vi "Z6CSMain.panel.vi"(0 "object ref":refnum<vi>, 5 "error in (no error)":errorcluster) -> (19 "error out":errorcluster)   [LabVIEW 2014, in "Z6CSMain.lvlib"]
doc: "This is just an example for a GUI thread.\n\nLicense Agreement for this software:\n\nCopyright (C)\nGesellschaft für Schwerionenforschung, GSI\nPlanckstr. 1\n64291 Darmstadt\nGermany\n\nContact: D.Beck@gsi.de \n\nThis program is free software; you can redistribute it and/or modify it under the terms of the GNU General Public License as published by the Free Software Foundation; either version 2 of the license, or (at your option) any later version.\n\nThis program is distributed in the hope that it will be useful, but WITHOUT ANYW ARRANTY; without even the implied warranty of MERCHANTABILITY or FITNESS FOR A PARTICULAR PURPOSE. See the GNU General License for more details (http://www.gnu.org).\n\nGesellschaft für Schwerionenforschung, GSI\nPlanckstr. 1, 64291 Darmstadt, Germany\nFor all questions and ideas contact: M.Richter@gsi.de, H.Brand@gsi.de or D.Beck@gsi.de.\nLast update: 18-DEC-2002"
uses:
  Z6CSMain.lvlib
  CS_Core/CSObj/CSObj.lvlib
  PH_Basics/PH_Common/PH_Common.lvlib
  PCSMain/PCSMain.lvlib
panel:
  in  "VISA":bool
  in  "Powermeter Statistician":bool
  in  "Powermeter List":bool
  in  "SHS Anal Statistician":bool
  in  "SHS Analyzer":bool
  in  "SHS Analysis Calibrator":bool
  in  "Remote Desktop Connection":bool
  in  "Minimize":bool
  in  "Beckhoff Watch Dog":bool
  in  "Countdown":bool
  in  "Seq Watch":bool
  in  "Vacuum Controllers":bool
  in  "SSAC":bool
  in  "Switch List":bool
  in  "BB List":bool
  in  "Spectrometer":bool
  in  "Z6 Beamline":bool
  in  "6P List":bool
  in  "Scopes":bool
  in  "Current Meas":bool
  in  "Calorimeter":bool
  in  "Cam List":bool
  in  "PCS System Indicator":bool caption="PCS"
  in  "Fast CoG":bool
  in  "Image Statistician":bool
  in  "Powermeter":bool
  in  "DataViewer":bool
  in  "Beamline":bool
  out "stopped":bool
  in  "BlackBoxes":bool
  in  "Operators":bool
  in  "Calibrator":bool
  in  "GateDelayGens":bool
  in  "Switch GUIs":bool
  in  "Motion GUIs":bool
  in  "Cameras":bool
  in  "Sequencer":bool
  in  "Delete":bool
  out "loop counter":i32
  # "Z6-CS"
  # "3.40"
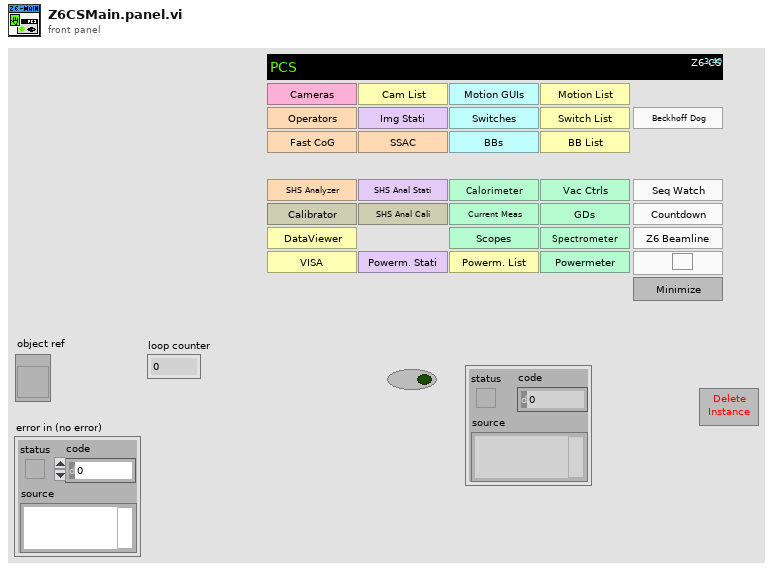
[diagram p1: front panel]
types:
  T1 = enum16{"None", "PCS Main", "Z6 Main", "PCS Beamline", "Z6 Beamline", "Image Statistician", "Powermeter Statistician", "SHS Anal Statistician", "Image Center of Gravity", "Image Calibrator", "SHS Analysis Calibrator"}
  T2 = enum16{"None", "PCS Main", "Z6 Main", "PCS Beamline", "Z6 Beamline", "Image Statistician", "Powermeter Statistician", "SHS Anal Statistician", "Image Center of Gravity", "Image Calibrator", "SHS Analysis Calibrator", "Cam List", "Powermeterlist", "6P List", "BB List", "Switch List", "Sequence Watch"}
  T3 = typedef "PCSMain.lvlib/PCSMain.i attribute.ctl" = cluster{"System Objects":cluster{"Spectrometer Objects":string[], "Camera Objects":string[], "Image Operator Objects":string[], "Gate- and Delaygenerators":string[], "Current Meas Objects":string[], "Calorimeter Objects":string[], "Powermeter Objects":string[], "SSAC Objects":string[], "Vacuum Control Objects":string[], "Countdown Counter Objects":string[], "Beckhoff Watchdog Objects":string[], "SHS Analyzer Objects":string[]}, "Local Objects":cluster{"Spectrometer Objects":string[], "Camera Objects":string[], "Image Operator Objects":string[], "Gate- and Delaygenerators":string[], "Current Meas Objects":string[], "Calorimeter Objects":string[], "Powermeter Objects":string[], "SSAC Objects":string[], "Vacuum Control Objects":string[], "Countdown Counter Objects":string[], "Beckhoff Watchdog Objects":string[], "SHS Analyzer Objects":string[]}, "Systems on same node":string[], "Data Viewer visible?":bool, "Running Objects":cluster{"Operators":bool, "SHS Analyzers":bool}, "Cam Instance System ID":string, "Black Box Objects":string[], "Switch Objects":string[], "Motion GUI Objects":string[], "Osci Objects":string[]}
  T4 = enum16{"PCS", "Laser", "Vision", "PP", "Special", "Beckhoff"}
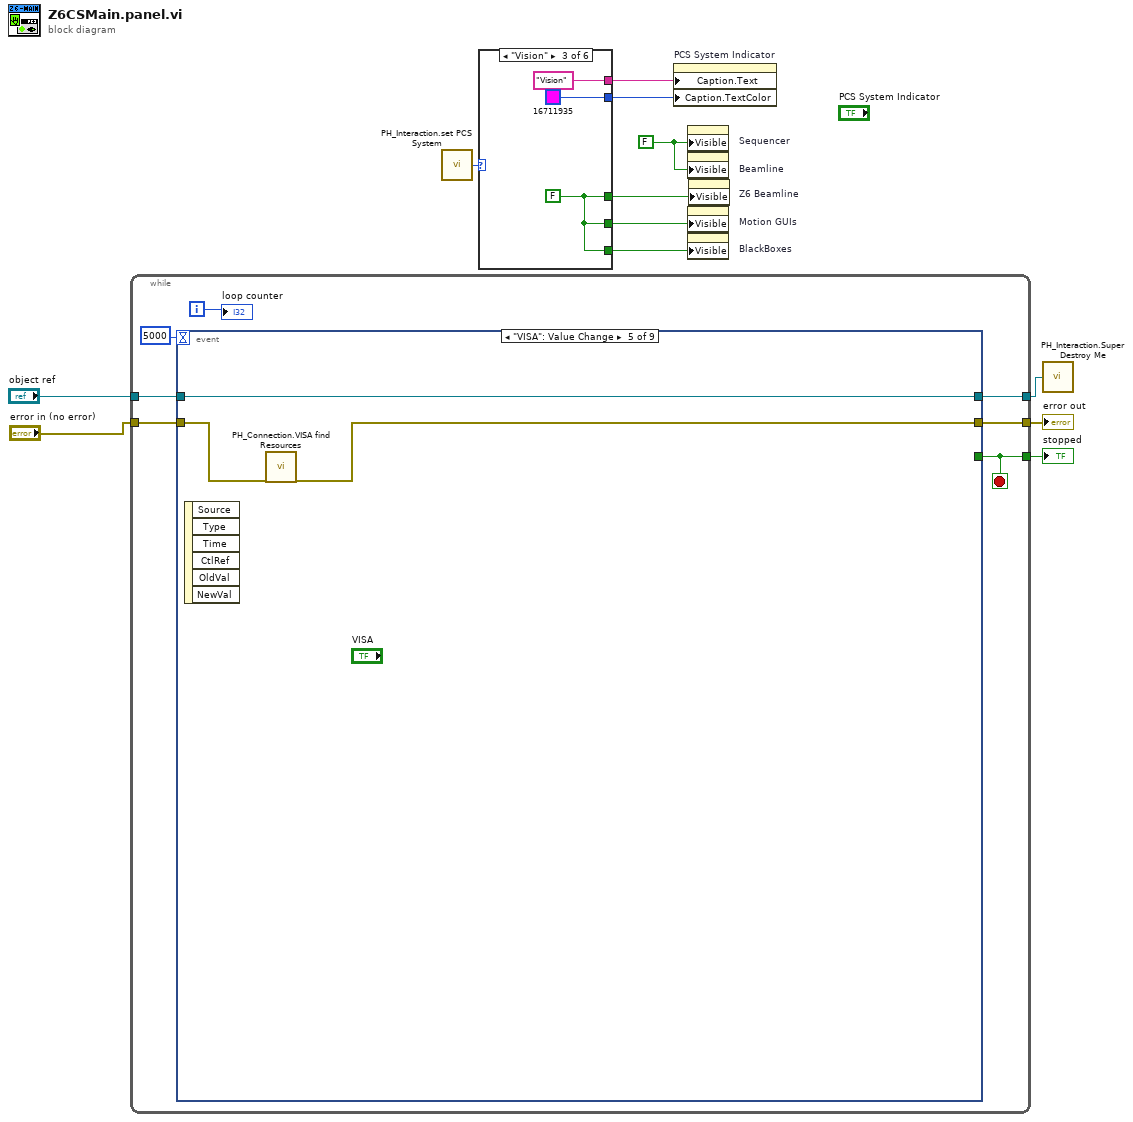
[diagram p0: block diagram]
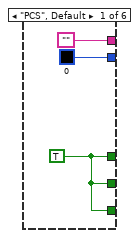
[diagram p2: hidden frame]
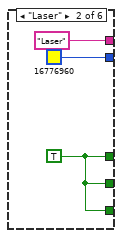
[diagram p3: hidden frame]
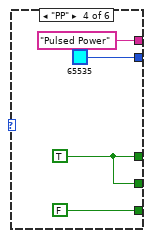
[diagram p4: hidden frame]
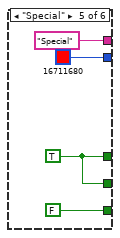
[diagram p5: hidden frame]
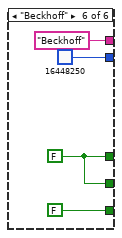
[diagram p6: hidden frame]
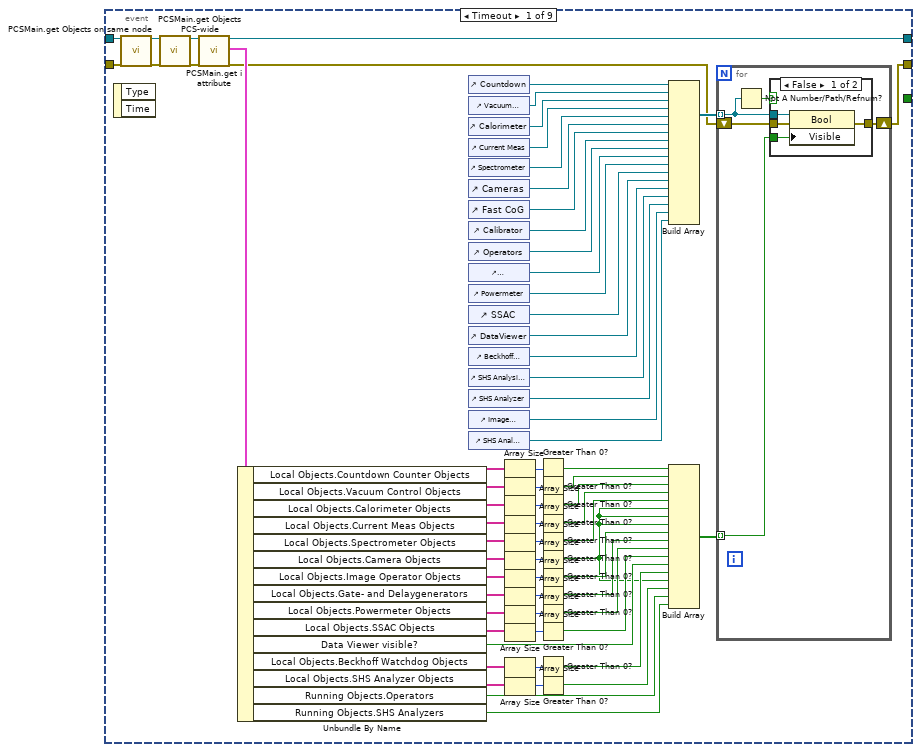
[diagram p7: hidden frame]
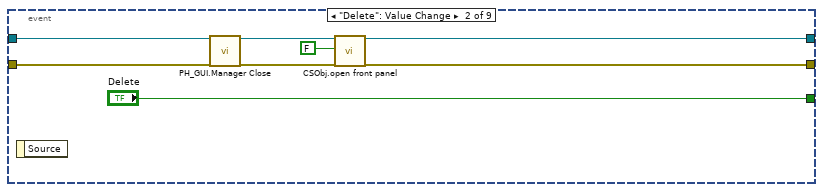
[diagram p9: hidden frame]
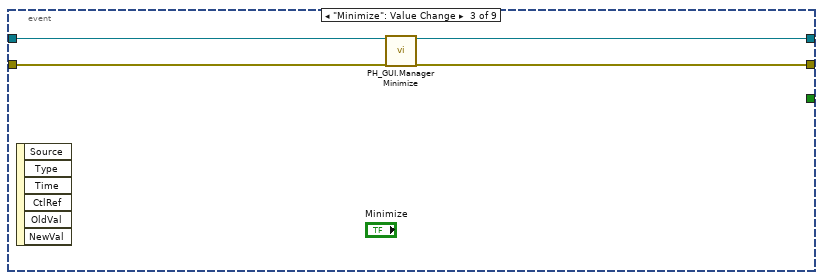
[diagram p10: hidden frame]
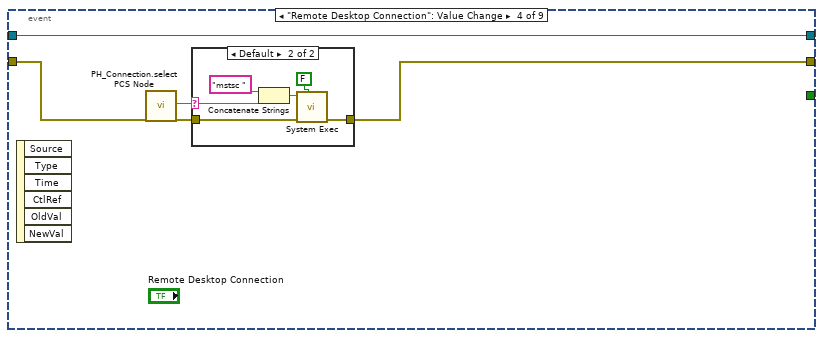
[diagram p11: hidden frame]
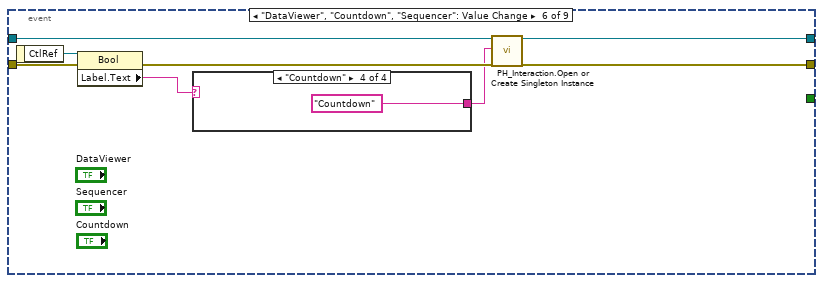
[diagram p13: hidden frame]
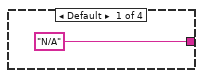
[diagram p14: hidden frame]
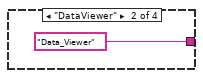
[diagram p15: hidden frame]
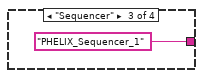
[diagram p16: hidden frame]
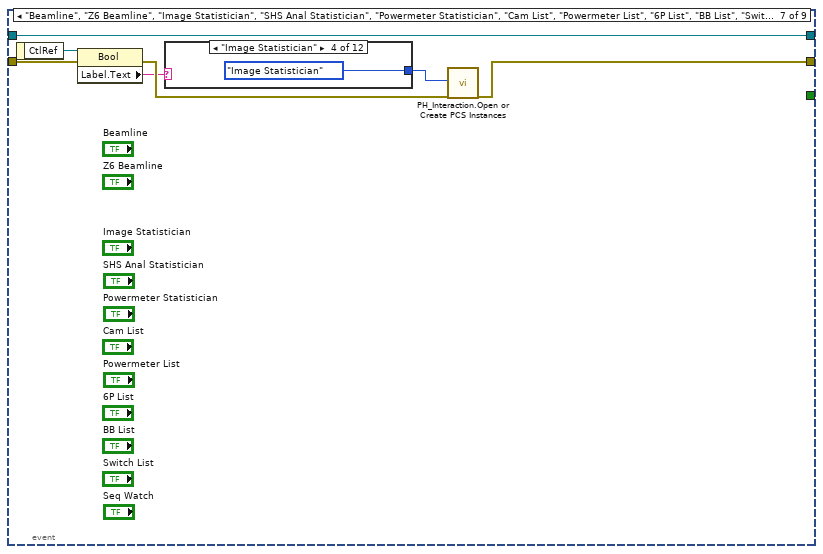
[diagram p17: hidden frame]
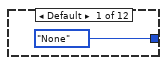
[diagram p18: hidden frame]
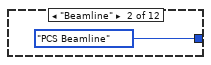
[diagram p19: hidden frame]
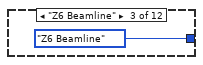
[diagram p20: hidden frame]
diagram:
  w1 = FALSE
  n1 = while {
    tunnel: "object ref" -> [w15]
    tunnel: [w14] -> w10
    tunnel: [w18] -> w11
    tunnel: "error in (no error)" -> [w17]
    tunnel: [w16] -> w12
    i -> [w19]
    stop <- w16 stop-if-true
    n2 = event shown="[4] \"VISA\": Value Change" {
      selector: _ -> [_ _ _ _ _ _ _ _ _]
      dyn-events: _ -> [_ _ _ _ _ _ _ _ _]
      timeout: 5000 -> [_ _ _ _ _ _ _ _ _]
      tunnel: w15 -> [w87 w104 w110 w114 w125 w128 w141 w164 w182]
      tunnel: [_ "Delete" _ _ _ _ _ _ _] -> w16
      tunnel: [w62 w103 w107 w112 w123 w129 w144 w167 w180] -> w18
      tunnel: w17 -> [w88 w100 w109 w115 w124 w132 w142 w165 w181]
      tunnel: [w61 w102 w108 w114 w125 w127 w141 w163 w176] -> w14
      event Timeout {
        n3 = event-data() -> ()  [unwired: 1 in, 2 out]
        n4 = call "PCSMain.get Objects on same node.vi"("i ref in"=w87, "error in (no error)"=w88) -> ("i ref out"=w23:refnum<vi>, "error out"=w21:errorcluster)  [unwired: 16 in]
        n5 = call "PCSMain.get Objects PCS-wide.vi"("i ref in"=w23, "error in (no error)"=w21) -> ("i ref out"=w22:refnum<vi>, "error out"=w20:errorcluster)  [unwired: 16 in]
        n6 = call "PCSMain.get i attribute.vi"("i ref in"=w22, "error in (no error)"=w20) -> ("i ref out"=w61:refnum<vi>, "i attribute"=w86:T3, "error out"=w63:errorcluster)  [unwired: 15 in]
        n7 = Unbundle By Name(w86) -> ("Local Objects.Countdown Counter Objects"=w43:string[], "Local Objects.Vacuum Control Objects"=w47:string[], "Local Objects.Calorimeter Objects"=w82:string[], "Local Objects.Current Meas Objects"=w75:string[], "Local Objects.Spectrometer Objects"=w73:string[], "Local Objects.Camera Objects"=w71:string[], "Local Objects.Image Operator Objects"=w70:string[], "Local Objects.Gate- and Delaygenerators"=w68:string[], "Local Objects.Powermeter Objects"=w66:string[], "Local Objects.SSAC Objects"=w38:string[], "Data Viewer visible?"=w49:bool, "Local Objects.Beckhoff Watchdog Objects"=w40:string[], "Local Objects.SHS Analyzer Objects"=w30:string[], "Running Objects.Operators"=w25:bool, "Running Objects.SHS Analyzers"=w24:bool)
        n8 = control-ref of="Countdown"() -> (w44:refnum<vi>)
        n9 = control-ref of="Vacuum Controllers"() -> (w48:refnum<vi>)
        n10 = control-ref of="Calorimeter"() -> (w60:refnum<vi>)
        n11 = control-ref of="Current Meas"() -> (w59:refnum<vi>)
        n12 = control-ref of="Spectrometer"() -> (w58:refnum<vi>)
        n13 = control-ref of="Cameras"() -> (w57:refnum<vi>)
        n14 = control-ref of="Fast CoG"() -> (w53:refnum<vi>)
        n15 = control-ref of="Calibrator"() -> (w52:refnum<vi>)
        n16 = control-ref of="Operators"() -> (w56:refnum<vi>)
        n17 = control-ref of="GateDelayGens"() -> (w55:refnum<vi>)
        n18 = control-ref of="Powermeter"() -> (w54:refnum<vi>)
        n19 = control-ref of="SSAC"() -> (w51:refnum<vi>)
        n20 = control-ref of="DataViewer"() -> (w50:refnum<vi>)
        n21 = control-ref of="Beckhoff Watch Dog"() -> (w35:refnum<vi>)
        n22 = control-ref of="SHS Analysis Calibrator"() -> (w33:refnum<vi>)
        n23 = control-ref of="SHS Analyzer"() -> (w28:refnum<vi>)
        n24 = control-ref of="Image Statistician"() -> (w27:refnum<vi>)
        n25 = control-ref of="SHS Anal Statistician"() -> (w26:refnum<vi>)
        n26 = Array Size(array=w43) -> (size(s)=w41:i32)
        n27 = Array Size(array=w47) -> (size(s)=w45:i32)
        n28 = Array Size(array=w82) -> (size(s)=w83:i32)
        n29 = Array Size(array=w75) -> (size(s)=w80:i32)
        n30 = Array Size(array=w73) -> (size(s)=w79:i32)
        n31 = Array Size(array=w71) -> (size(s)=w78:i32)
        n32 = Array Size(array=w70) -> (size(s)=w77:i32)
        n33 = Array Size(array=w68) -> (size(s)=w76:i32)
        n34 = Array Size(array=w66) -> (size(s)=w64:i32)
        n35 = Array Size(array=w38) -> (size(s)=w37:i32)
        n36 = Array Size(array=w40) -> (size(s)=w39:i32)
        n37 = Array Size(array=w30) -> (size(s)=w31:i32)
        n38 = Greater Than 0?(x=w41) -> (x > 0?=w42:bool)
        n39 = Greater Than 0?(x=w45) -> (x > 0?=w46:bool)
        n40 = Greater Than 0?(x=w83) -> (x > 0?=w81:bool)
        n41 = Greater Than 0?(x=w80) -> (x > 0?=w74:bool)
        n42 = Greater Than 0?(x=w79) -> (x > 0?=w72:bool)
        n43 = Greater Than 0?(x=w78) -> (x > 0?=w32:bool)
        n44 = Greater Than 0?(x=w77) -> (x > 0?=w69:bool)
        n45 = Greater Than 0?(x=w76) -> (x > 0?=w67:bool)
        n46 = Greater Than 0?(x=w64) -> (x > 0?=w65:bool)
        n47 = Greater Than 0?(x=w37) -> (x > 0?=w36:bool)
        n48 = Greater Than 0?(x=w39) -> (x > 0?=w34:bool)
        n49 = Greater Than 0?(x=w31) -> (x > 0?=w29:bool)
        n50 = Build Array(w44, w48, w60, w59, w58, w57, w53, w52, w56, w55, w54, w51, w50, w35, w33, w28, w27, w26) -> (w85:refnum<vi>[])
        n51 = Build Array(w42, w46, w81, w74, w72, w32, w32, w32, w69, w67, w65, w36, w49, w34, w32, w29, w25, w24) -> (w84:bool[])
        n52 = for {
          tunnel: w84 -> [w89] mode=indexing
          tunnel: w85 -> [w92] mode=indexing
          shift-right: [w91] -> w62
          shift-left: w63 -> [w90]
          n53 = Not A Number/Path/Refnum?(number/path/refnum=w92) -> (NaN/Path/Refnum?=w93:bool)
          n54 = case shown="False" w93 {
            tunnel: w89 -> [w97 _]
            tunnel: w92 -> [w96 _]
            tunnel: w90 -> [w95 w98]
            tunnel: [w94 w98] -> w91
            frame False {
              n55 = property class="Bool"(reference=w96, error in=w95, "Visible"=w97) -> (error out=w94:errorcluster)  [unwired: 1 out]
            }
            frame True {
            }
          }
        }
      }
      event "Delete": Value Change {
        n56 = event-data() -> ()  [unwired: 1 in, 1 out]
        n57 = call "PH_GUI.Manager Close.vi"("i ref in"=w104, "error in"=w100) -> ("i ref out"=w101:refnum<vi>, "error out"=w99:errorcluster)  [unwired: 16 in]
        n58 = call "CSObj.open front panel.vi"("i ref in"=w101, "frontPanelOpen"=FALSE ("front panel open"), "error in (no error)"=w99) -> ("i ref out"=w102:refnum<vi>, "error out"=w103:errorcluster)  [unwired: 15 in]
      }
      event "Minimize": Value Change {
        n59 = event-data() -> ()  [unwired: 1 in, 6 out]
        n60 = call "PH_GUI.Manager Minimize.vi"("i ref in"=w110, "error in"=w109) -> ("i ref out"=w108:refnum<vi>, "error out"=w107:errorcluster)  [unwired: 16 in]
      }
      event "Remote Desktop Connection": Value Change {
        n61 = event-data() -> ()  [unwired: 1 in, 6 out]
        n62 = call "PH_Connection.select PCS Node.vi"("error in"=w115) -> ("string out"=w111:string, "error out"=w113:errorcluster)  [unwired: 17 in]
        n63 = case shown="Default" w111 {
          selector: w111 -> [_ w117]
          tunnel: w113 -> [w116 w119]
          tunnel: [w116 w118] -> w112
          frame "", "N/A" {
          }
          frame Default {
            n64 = Concatenate Strings("mstsc " ("command line"), w117) -> (w121:string)
            n65 = call <vilib>:"System Exec.vi"("wait until completion? (T)"=FALSE, "error in (no error)"=w119, "command line"=w121) -> ("error out"=w118:errorcluster)  [unwired: 5 in, 3 out]
          }
        }
      }
      event "VISA": Value Change {
        n66 = event-data() -> ()  [unwired: 1 in, 6 out]
        n67 = call "PH_Connection.VISA find Resources.vi"("error in"=w124) -> ("error out"=w123:errorcluster)  [unwired: 17 in, 1 out]
      }
      event "DataViewer", "Countdown", "Sequencer": Value Change {
        n68 = event-data() -> ("CtlRef"=w133:refnum<vi>)  [unwired: 1 in]
        n69 = property class="Bool"(reference=w133, error in=w132) -> (error out=w130:errorcluster, "Label.Text"=w131:string)  [unwired: 1 out]
        n70 = case shown="\"Countdown\"" w131 {
          tunnel: ["N/A" "Data_Viewer" "PHELIX_Sequencer_1" "Countdown"] -> w126
          frame Default {
          }
          frame "DataViewer" {
          }
          frame "Sequencer" {
          }
          frame "Countdown" {
          }
        }
        n71 = call "PH_Interaction.Open or Create Singleton Instance.vi"("i ref in"=w128, "Instance to create or to open"=w126, "error IO"=w130) -> ("i ref out"=w127:refnum<vi>, "error out"=w129:errorcluster)  [unwired: 15 in]
      }
      event "Beamline", "Z6 Beamline", "Image Statistician", "SHS Anal Statistician", "Powermeter Statistician", "Cam List", "Powermeter List", "6P List", "BB List", "Switch List", "Seq Watch": Value Change {
        n72 = event-data() -> ("CtlRef"=w143:refnum<vi>)  [unwired: 1 in]
        n73 = property class="Bool"(reference=w143, error in=w142) -> (error out=w140:errorcluster, "Label.Text"=w139:string)  [unwired: 1 out]
        n74 = case shown="\"Image Statistician\"" w139 {
          tunnel: [T1."None" ("Instance to create or open") T1."PCS Beamline" ("Instance to create or open") T1."Z6 Beamline" ("Instance to create or open") T1."Image Statistician" ("Instance to create or open") T1."SHS Anal Statistician" ("Instance to create or open") T1."Powermeter Statistician" ("Instance to create or open") T2."Cam List" ("Instance to create or open") T2."Powermeterlist" ("Instance to create or open") T2."6P List" ("Instance to create or open") T2."BB List" ("Instance to create or open") T2."Switch List" ("Instance to create or open") T2."Sequence Watch" ("Instance to create or open")] -> w138
          frame Default {
          }
          frame "Beamline" {
          }
          frame "Z6 Beamline" {
          }
          frame "Image Statistician" {
          }
          frame "SHS Anal Statistician" {
          }
          frame "Powermeter Statistician" {
          }
          frame "Cam List" {
          }
          frame "Powermeter List" {
          }
          frame "6P List" {
          }
          frame "BB List" {
          }
          frame "Switch List" {
          }
          frame "Seq Watch" {
          }
        }
        n75 = call "PH_Interaction.Open or Create PCS Instances.vi"("Instance to create or open"=w138, "error IO"=w140) -> ("error out"=w144:errorcluster)  [unwired: 17 in]
      }
      event "Calibrator", "SHS Analysis Calibrator", "Fast CoG": Value Change {
        n76 = event-data() -> ("CtlRef"=w166:refnum<vi>)  [unwired: 1 in]
        n77 = property class="Bool"(reference=w166, error in=w165) -> (error out=w162:errorcluster, "Label.Text"=w158:string)  [unwired: 1 out]
        n78 = case shown="\"Fast CoG\"" w158 {
          tunnel: [T1."None" ("Instance to create or open") T1."Image Calibrator" ("Instance to create or open") T1."SHS Analysis Calibrator" ("Instance to create or open") T1."Image Center of Gravity" ("Instance to create or open")] -> w157
          frame Default {
          }
          frame "Calibrator" {
          }
          frame "SHS Analysis Calibrator" {
          }
          frame "Fast CoG" {
          }
        }
        n79 = call "PCSMain.get i attribute.vi"("i ref in"=w164, "error in (no error)"=w162) -> ("i ref out"=w163:refnum<vi>, "i attribute"=w160:T3, "error out"=w161:errorcluster)  [unwired: 15 in]
        n80 = Unbundle By Name(w160) -> ("Cam Instance System ID"=w159:string)
        n81 = call "PH_Interaction.Open or Create PCS Instances.vi"("System ID (N/A)"=w159, "Instance to create or open"=w157, "error IO"=w161) -> ("error out"=w167:errorcluster)  [unwired: 16 in]
      }
      event "Spectrometer", "Cameras", "Operators", "GateDelayGens", "Current Meas", "Calorimeter", "Powermeter", "SSAC", "Vacuum Controllers", "Beckhoff Watch Dog", "SHS Analyzer", "Switch GUIs", "BlackBoxes", "Motion GUIs", "Scopes": Value Change {
        n82 = event-data() -> ("CtlRef"=w178:refnum<vi>)  [unwired: 1 in]
        n83 = property class="Bool"(reference=w178) -> ("Label.Text"=w175:string)  [unwired: 1 in, 2 out]
        n84 = call "PCSMain.get i attribute.vi"("i ref in"=w182, "error in (no error)"=w181) -> ("i ref out"=w177:refnum<vi>, "i attribute"=w174:T3, "error out"=w179:errorcluster)  [unwired: 15 in]
        n85 = case shown="\"Vacuum Controllers\"" w175 {
          tunnel: w174 -> [_ w190 w193 w196 w199 w202 w205 w208 w211 w214 w217 w220 w223 w226 w229 w232]
          tunnel: [string[] [] ("Spectrometer Objects") w189 w191 w194 w197 w200 w204 w207 w210 w213 w216 w219 w222 w225 w228 w231] -> w173
          tunnel: ["N/A" ("Caption.Text") "Spectrometer" ("Caption.Text") "Switch GUIs" ("Caption.Text") "Black Boxes" ("Caption.Text") "Motion GUIs" ("Caption.Text") "Oscilloscopes" ("Caption.Text") "Cameras" ("Caption.Text") "Image Operators" ("Caption.Text") "SHS Analyzers" ("Caption.Text") "Gate and Delay Generators" ("Caption.Text") "Current Measurement" ("Caption.Text") "Calorimeter" ("Caption.Text") "Powermeter" ("Caption.Text") "SSAC" ("Caption.Text") "Vacuum Controller" ("Caption.Text") "Beckhoff Watchdog" ("Caption.Text")] -> w172
          frame Default {
          }
          frame "Spectrometer" {
            n86 = Unbundle By Name(w190) -> ("Local Objects.Spectrometer Objects"=w189:string[])
          }
          frame "Switch GUIs" {
            n87 = Unbundle By Name(w193) -> ("Switch Objects"=w191:string[])
          }
          frame "BlackBoxes" {
            n88 = Unbundle By Name(w196) -> ("Black Box Objects"=w194:string[])
          }
          frame "Motion GUIs" {
            n89 = Unbundle By Name(w199) -> ("Motion GUI Objects"=w197:string[])
          }
          frame "Scopes" {
            n90 = Unbundle By Name(w202) -> ("Osci Objects"=w200:string[])
          }
          frame "Cameras" {
            n91 = Unbundle By Name(w205) -> ("Local Objects.Camera Objects"=w204:string[])
          }
          frame "Operators" {
            n92 = Unbundle By Name(w208) -> ("Local Objects.Image Operator Objects"=w207:string[])
          }
          frame "SHS Analyzer" {
            n93 = Unbundle By Name(w211) -> ("Local Objects.SHS Analyzer Objects"=w210:string[])
          }
          frame "GateDelayGens" {
            n94 = Unbundle By Name(w214) -> ("Local Objects.Gate- and Delaygenerators"=w213:string[])
          }
          frame "Current Meas" {
            n95 = Unbundle By Name(w217) -> ("Local Objects.Current Meas Objects"=w216:string[])
          }
          frame "Calorimeter" {
            n96 = Unbundle By Name(w220) -> ("Local Objects.Calorimeter Objects"=w219:string[])
          }
          frame "Powermeter" {
            n97 = Unbundle By Name(w223) -> ("Local Objects.Powermeter Objects"=w222:string[])
          }
          frame "SSAC" {
            n98 = Unbundle By Name(w226) -> ("Local Objects.SSAC Objects"=w225:string[])
          }
          frame "Vacuum Controllers" {
            n99 = Unbundle By Name(w229) -> ("Local Objects.Vacuum Control Objects"=w228:string[])
          }
          frame "Beckhoff Watch Dog" {
            n100 = Unbundle By Name(w232) -> ("Local Objects.Beckhoff Watchdog Objects"=w231:string[])
          }
        }
        n101 = call "PH_Strings.select string from array.vi"("String Array in"=w173, "Caption.Text"=w172, "error in (no error)"=w179) -> ("string out"=w185:string, "index"=w183:i32, "error out"=w184:errorcluster)  [unwired: 14 in]
        n102 = case shown="-1" w183 {
          tunnel: w184 -> [w234 w239]
          tunnel: [w234 w238] -> w180
          tunnel: w185 -> [_ w237]
          tunnel: w177 -> [w233 w236]
          tunnel: [w233 w235] -> w176
          frame -1 {
          }
          frame Default {
            n103 = call "PH_Interaction.Open or Create Singleton Instance.vi"("i ref in"=w236, "Instance to create or to open"=w237, "error IO"=w239) -> ("i ref out"=w235:refnum<vi>, "error out"=w238:errorcluster)  [unwired: 15 in]
          }
        }
      }
    }
    "loop counter" <- w19
  }
  "error out" <- w11
  "stopped" <- w12
  n104 = call "PH_Interaction.set PCS System.vi"() -> ("Enum"=w9:T4)  [unwired: 1 in]
  n105 = case shown="\"Vision\"" w9 {
    tunnel: ["" "Laser" "Vision" "Pulsed Power" "Special" "Beckhoff"] -> w8
    tunnel: [w241 w244 w247 w251 w255 w259] -> w7
    tunnel: [w241 w244 w247 FALSE FALSE FALSE] -> w6
    tunnel: [w241 w244 w247 w251 w255 w259] -> w5
    tunnel: [u32 0 ("Color Box") u32 16776960 ("Color Box") u32 16711935 ("Color Box") u32 65535 ("Color Box") u32 16711680 ("Color Box") u32 16448250 ("Color Box")] -> w2
    frame "PCS", Default {
      w241 = TRUE
    }
    frame "Laser" {
      w244 = TRUE
    }
    frame "Vision" {
      w247 = FALSE
    }
    frame "PP" {
      w251 = TRUE
    }
    frame "Special" {
      w255 = TRUE
    }
    frame "Beckhoff" {
      w259 = FALSE
    }
  }
  n106 = property on="PCS System Indicator" class="Bool (strict)"("Caption.Text"=w8, "Caption.TextColor"=w2) -> ()  [unwired: 2 in, 2 out]
  n107 = property on="Sequencer" class="Bool"("Visible"=w1) -> ()  [unwired: 2 in, 2 out]
  n108 = property on="Beamline" class="Bool"("Visible"=w1) -> ()  [unwired: 2 in, 2 out]
  n109 = property on="Motion GUIs" class="Bool"("Visible"=w7) -> ()  [unwired: 2 in, 2 out]
  n110 = property on="BlackBoxes" class="Bool"("Visible"=w6) -> ()  [unwired: 2 in, 2 out]
  n111 = property on="Z6 Beamline" class="Bool"("Visible"=w5) -> ()  [unwired: 2 in, 2 out]
  n112 = call "PH_Interaction.Super Destroy Me.vi"("i ref out"=w10) -> ()
